vi "HCC Agilent Tester.vi"() -> ()   [LabVIEW 2016]
uses:
  Agilent 34970.lvlib
panel:
  in  "error in (no error)":errorcluster
  out "error out":errorcluster
  in  "VISA Resource Name":refnum<visa-resource-name>
  in  "stop":bool
  out "Unsorted Data":dbl[](array[numeric]) format="%.2f"
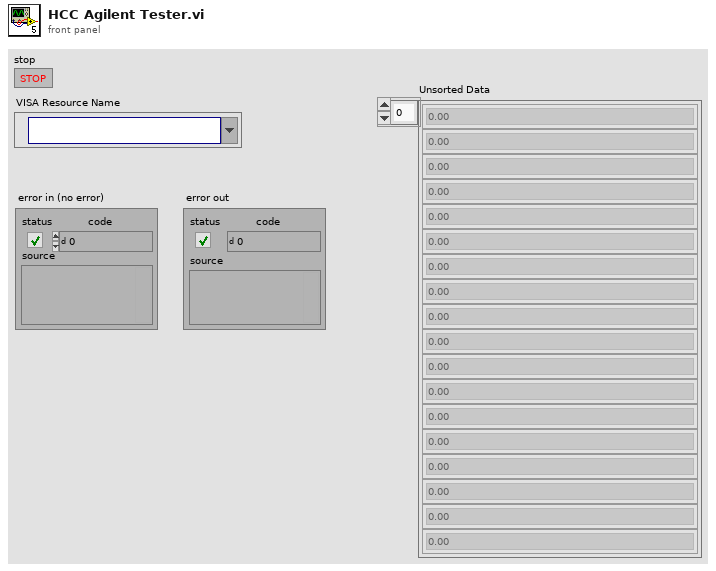
[diagram p1: front panel]
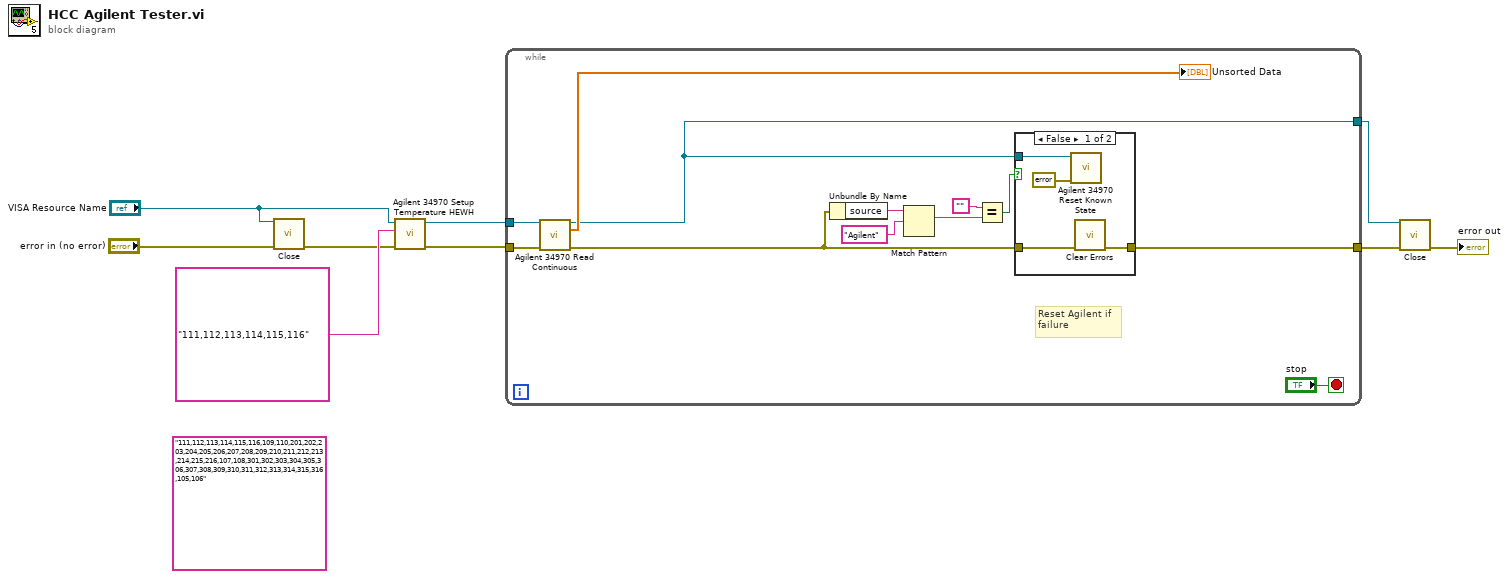
[diagram p0: block diagram]
diagram:
  (unwired) "111,112,113,114,115,116,109,110,201,202,203,204,205,206,207,208,209,210,211,212,213,214,215,216,107,108,301,302,303,304,305,306,307,308,309,310,311,312,313,314,315,316,105,106" ("Agilent Channel Input")
  n1 = call "Close.vi"("VISA Resource Name"="VISA Resource Name", "error in (no error)"="error in (no error)") -> ("error out"=w3:errorcluster)  [unwired: 13 in]
  n2 = call "Agilent 34970 Setup Temperature HEWH.vi"("Error In"=w3, "Agilent Channel Input"="111,112,113,114,115,116", "VISA Refnum in"="VISA Resource Name") -> ("Error Out"=w8:errorcluster, "VISA Resource Name Out"=w9:refnum<visa-resource-name>)  [unwired: 7 in]
  n3 = while {
    tunnel: w8 -> [w15]
    tunnel: w9 -> [w14]
    tunnel: [w13] -> w6
    tunnel: [w10] -> w5
    stop <- "stop" stop-if-true
    # "Reset Agilent if \nfailure"
    n4 = call "Agilent 34970 Read Continuous.vi"("VISA Resource Name"=w14, "error in (no error)"=w15) -> ("VISA resource name out"=w10:refnum<visa-resource-name>, "Output Array"=→"Unsorted Data":dbl[], "error out"=w11:errorcluster)  [unwired: 10 in, 1 out]
    n5 = Unbundle By Name(w11) -> ("source"=w21:string)
    n6 = Match Pattern(string=w21, regular expression="Agilent") -> (match substring=w17:string)  [unwired: 1 in, 3 out]
    n7 = Equal?(x="", y=w17) -> (x = y?=w19:bool)
    n8 = case shown="False" w19 {
      tunnel: w11 -> [w23 w26]
      tunnel: [w22 w26] -> w13
      tunnel: w10 -> [w24 _]
      frame False {
        n9 = call "Agilent 34970 Reset Known State.vi"("Error In"=errorcluster {"status"=TRUE, "code"=0, "source"=""}, "VISA Refnum in"=w24) -> ()  [unwired: 9 in, 1 out]
        n10 = call <vilib>:"Clear Errors.vi"("error in (no error)"=w23) -> ("error out"=w22:errorcluster)  [unwired: 5 in, 1 out]
      }
      frame True {
      }
    }
  }
  n11 = call "Close.vi"("VISA Resource Name"=w5, "error in (no error)"=w6) -> ("error out"=→"error out":errorcluster)  [unwired: 13 in]
